vi "RegSaveTemp.vi"() -> ()   [LabVIEW 2012]
panel:
  out "I7":bool
  out "I6":bool
  out "I5":bool
  out "I4":bool
  out "I3":bool
  out "I2":bool
  out "I1":bool
  out "I0":bool
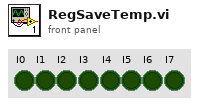
[diagram p1: front panel]
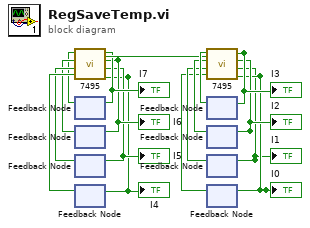
[diagram p0: block diagram]
diagram:
  n1 = feedback #1() -> (w10:bool)  [unwired: 1 in]
  n2 = feedback #2() -> (w11:bool)  [unwired: 1 in]
  n3 = feedback #3() -> (w12:bool)  [unwired: 1 in]
  n4 = feedback #4() -> (w13:bool)  [unwired: 1 in]
  n5 = call "7495.vi"("D"=w13, "C"=w12, "B"=w11, "A"=w10) -> ("OD"=w1:bool, "OC"=w5:bool, "OB"=w7:bool, "OA"=w8:bool, "Mode\nControl"=w9:bool)  [unwired: 3 in]
  "I4" <- w1
  "I5" <- w5
  "I6" <- w7
  "I7" <- w8
  n6 = feedback-in #1(w8) -> ()
  n7 = feedback-in #2(w7) -> ()
  n8 = feedback-in #3(w5) -> ()
  n9 = feedback-in #4(w1) -> ()
  n10 = feedback #5() -> (w17:bool)  [unwired: 1 in]
  n11 = feedback #6() -> (w16:bool)  [unwired: 1 in]
  n12 = feedback #7() -> (w15:bool)  [unwired: 1 in]
  n13 = feedback #8() -> (w14:bool)  [unwired: 1 in]
  n14 = call "7495.vi"("Mode\nControl"=w9, "D"=w14, "C"=w15, "B"=w16, "A"=w17) -> ("OD"=w3:bool, "OC"=w2:bool, "OB"=w4:bool, "OA"=w6:bool)  [unwired: 3 in]
  "I0" <- w3
  "I1" <- w2
  "I2" <- w4
  "I3" <- w6
  n15 = feedback-in #5(w6) -> ()
  n16 = feedback-in #6(w4) -> ()
  n17 = feedback-in #7(w2) -> ()
  n18 = feedback-in #8(w3) -> ()
